vi "Cria_arquivo_config.vi"(8 "error in (no error)":errorcluster, 11 "refnum in":path) -> (0 "error out":errorcluster, 3 "refnum":T1)   [LabVIEW 2019]
uses:
  <vilib>/Utility/config.llb/Config Data RefNum.ctl
  <vilib>/Utility/config.llb/Write Key (String).vi
  <vilib>/Utility/config.llb/Write Key (Double).vi
  <vilib>/Utility/config.llb/NI_LVConfig.lvlib
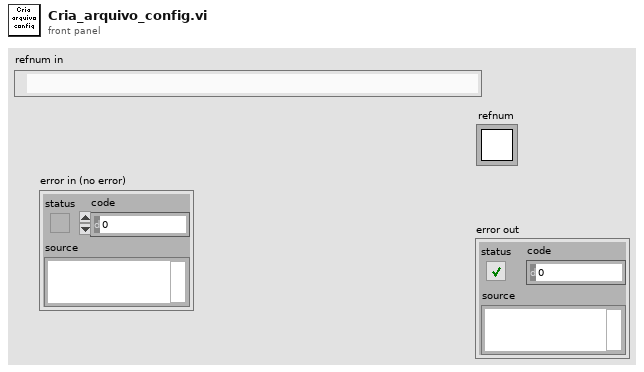
[diagram p1: front panel]
types:
  T1 = typedef "NI_LVConfig.lvlib/Config Data RefNum.ctl" = refnum<k1>
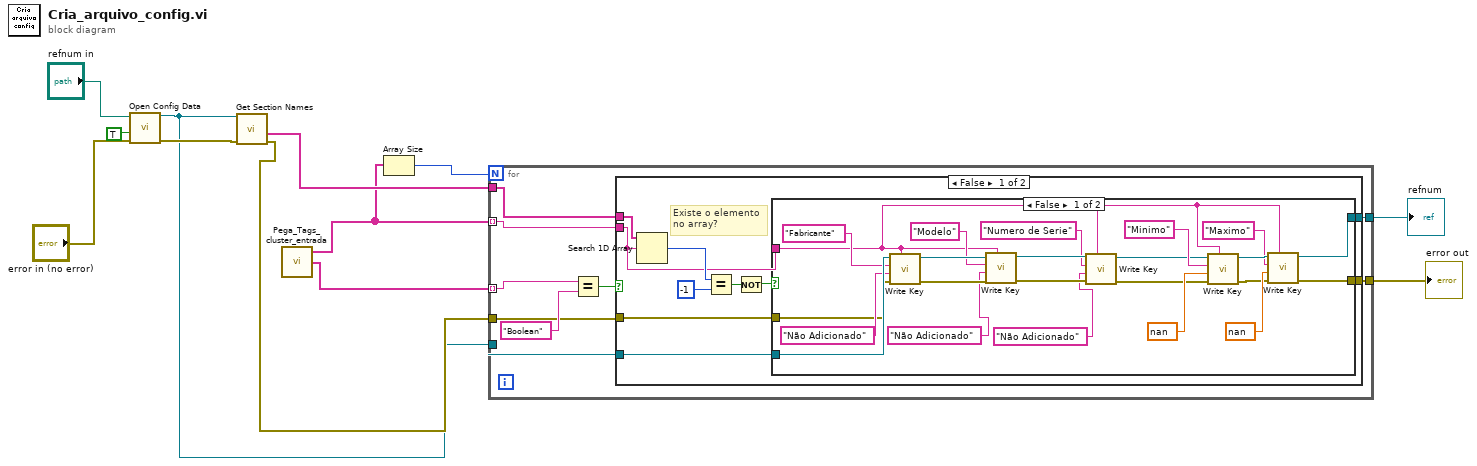
[diagram p0: block diagram]
diagram:
  n1 = call <vilib>:"Open Config Data.vi"("error in (no error)"="error in (no error)", "create file if necessary (T)"=TRUE, "configuration file path"="refnum in") -> ("error out"=w11:errorcluster, "refnum"=w6:T1)  [unwired: 6 in, 1 out]
  n2 = call <vilib>:"Get Section Names.vi"("error in (no error)"=w11, "refnum"=w6) -> ("error out"=w7:errorcluster, "section names"=w10:string[])  [unwired: 7 in, 1 out]
  n3 = call "Pega_Tags_cluster_entrada.vi"() -> ("TipoVariavel"=w5:string[], "Array Tags"=w9:string[])  [unwired: 4 in]
  n4 = Array Size(array=w9) -> (size(s)=w8:i32)
  n5 = for {
    N: w8 -> [_]
    tunnel: w9 -> [w18] mode=indexing
    tunnel: w10 -> [w17]
    tunnel: w7 -> [w15]
    tunnel: w6 -> [w16]
    tunnel: w5 -> [w20] mode=indexing
    tunnel: [w14] -> w2
    tunnel: [w13] -> w1
    n6 = Equal?(x=w20, y="Boolean") -> (x = y?=w19:bool)
    n7 = case shown="False" w19 {
      tunnel: w18 -> [w26 _]
      tunnel: w17 -> [w29 _]
      tunnel: w16 -> [w25 w57]
      tunnel: w15 -> [w24 w58]
      tunnel: [w23 w58] -> w14
      tunnel: [w22 w57] -> w13
      frame False {
        # "Existe o elemento\nno array?"
        n8 = Search 1D Array(1D array=w29, element=w26) -> (index of element=w28:i32)  [unwired: 1 in]
        n9 = Equal?(x=w28, y=-1) -> (x = y?=w31:bool)
        n10 = Not(x=w31) -> (.not. x?=w27:bool)
        n11 = case shown="False" w27 {
          tunnel: w26 -> [w34 _]
          tunnel: w25 -> [w54 w55]
          tunnel: w24 -> [w45 w56]
          tunnel: [w33 w56] -> w23
          tunnel: [w32 w55] -> w22
          frame False {
            n12 = call-poly <vilib>:"Write Key.vi"("section"=w34, "error in (no error)"=w45, "value"="Não Adicionado", "key"="Fabricante", "refnum"=w54) -> ("error out"=w41:errorcluster, "refnum out"=w44:T1)  [unwired: 4 in, 1 out]
            n13 = call-poly <vilib>:"Write Key.vi"("section"=w34, "error in (no error)"=w41, "value"="Não Adicionado", "key"="Modelo", "refnum"=w44) -> ("error out"=w40:errorcluster, "refnum out"=w43:T1)  [unwired: 4 in, 1 out]
            n14 = call-poly <vilib>:"Write Key.vi"("section"=w34, "error in (no error)"=w40, "value"="Não Adicionado", "key"="Numero de Serie", "refnum"=w43) -> ("error out"=w39:errorcluster, "refnum out"=w42:T1)  [unwired: 4 in, 1 out]
            n15 = call-poly <vilib>:"Write Key.vi"("section"=w34, "error in (no error)"=w39, "value"=nan, "key"="Minimo", "refnum"=w42) -> ("error out"=w46:errorcluster, "refnum out"=w53:T1)  [unwired: 4 in, 1 out]
            n16 = call-poly <vilib>:"Write Key.vi"("section"=w34, "error in (no error)"=w46, "value"=nan, "key"="Maximo", "refnum"=w53) -> ("error out"=w33:errorcluster, "refnum out"=w32:T1)  [unwired: 4 in, 1 out]
          }
          frame True {
          }
        }
      }
      frame True {
      }
    }
  }
  "error out" <- w2
  "refnum" <- w1
